vi "dfd_Super Narrowband Filter Design Convert to New Ripple.vi"(8 "ripple specs in":T1, 11 "new filter type":T2(ring)) -> (0 "ripple specs out":T1)   [LabVIEW 2017, in "NI_DigFilter_Process.lvlib"]
doc: "Converts the input ripple specification according to the type of narrowband filter."
uses:
  <vilib>/addons/Digital Filter Design/NI_DigFilter_Process.lvlib
  <vilib>/addons/Digital Filter Design/_Objects.llb/DFD Filter Ripple Specification (Design).ctl
  <vilib>/addons/Digital Filter Design/NI_DigFilter_Design.lvlib
  <vilib>/addons/Digital Filter Design/NI_DigFilterLicensed.lvlib
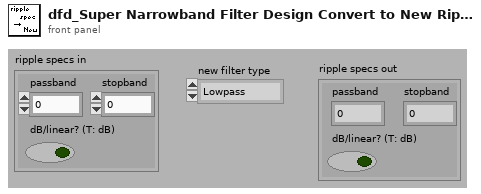
[diagram p1: front panel]
types:
  T1 = typedef "NI_DigFilterLicensed.lvlib/DFD Filter Ripple Specification (Design).ctl" = cluster{"passband":dbl, "stopband":dbl, "dB/linear? (T: dB)":bool}
  T2 = enum32{"Lowpass", "Highpass", "Bandpass", "Bandstop", "Wideband-Lowpass", "Wideband-Highpass"}
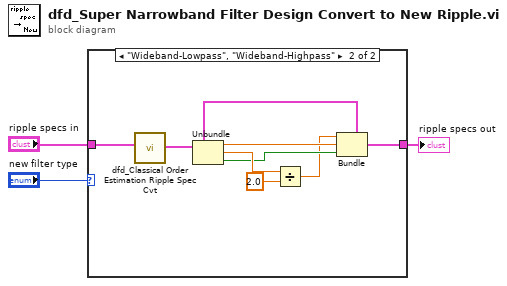
[diagram p0: block diagram]
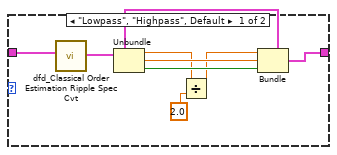
[diagram p2: hidden frame]
diagram:
  n1 = case shown="\"Wideband-Lowpass\", \"Wideband-Highpass\"" "new filter type" {
    tunnel: "ripple specs in" -> [w10 w18]
    tunnel: [w11 w19] -> w1
    frame "Lowpass", "Highpass", Default {
      n2 = call <vilib>:"dfd_Classical Order Estimation Ripple Spec Cvt.vi"("ripple specs"=w10) -> ("ripple specs (linear)"=w8:T1)  [unwired: 10 out]
      n3 = Unbundle(w8) -> ("passband"=w6:dbl, "stopband"=w7:dbl, "dB/linear? (T: dB)"=w9:bool)
      n4 = Divide(x=w6, y=2.0) -> (x/y=w4:dbl)
      n5 = Bundle(cluster=w8, "passband"=w4, "stopband"=w7, "dB/linear? (T: dB)"=w9) -> (w11:T1)
    }
    frame "Wideband-Lowpass", "Wideband-Highpass" {
      n6 = call <vilib>:"dfd_Classical Order Estimation Ripple Spec Cvt.vi"("ripple specs"=w18) -> ("ripple specs (linear)"=w14:T1)  [unwired: 10 out]
      n7 = Unbundle(w14) -> ("passband"=w17:dbl, "stopband"=w16:dbl, "dB/linear? (T: dB)"=w15:bool)
      n8 = Divide(x=w16, y=2.0) -> (x/y=w13:dbl)
      n9 = Bundle(cluster=w14, "passband"=w13, "stopband"=w17, "dB/linear? (T: dB)"=w15) -> (w19:T1)
    }
  }
  "ripple specs out" <- w1
